vi "Poisson CDF.vi"(10 "lambda":dbl=1.0, 11 "x":dbl=1.0) -> (0 "error":i32, 3 "cdf(x)":dbl=0.7357588823428847)   [LabVIEW 2010, in "NI_Gmath.lvlib"]
doc: "Computes the discrete cumulative distribution function (CDF), or the probability that the random variate X, where X describes the selected distribution type, takes on a value less than or equal to <B>x</B>. You must manually select the polymorphic instance to use."
uses:
  NI_Gmath.lvlib
panel:
  # "Poisson CDF"
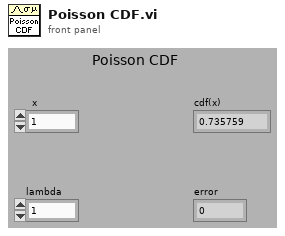
[diagram p1: front panel]
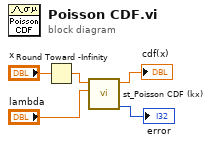
[diagram p0: block diagram]
diagram:
  n1 = Round Toward -Infinity(1:"x") -> (0:w1:dbl)
  n2 = call "st_Poisson CDF (kx).vi"("a"="lambda", "x"=w1) -> ("error"=→"error":i32, "cdf(x)"=→"cdf(x)":dbl)  [unwired: 8 in]
